vi "Configure Measurement (TOI - Tune Frequency).vi"(0 "VISA resource name":refnum<visa-resource-name>, 1 "Auto Upper Tune Frequency (T: Enable)":bool=TRUE, 2 "Manual Upper Tune Frequency  (2E+7 Hz)":dbl=20000000.0, 11 "error in (no error)":errorcluster, 12 "Auto Lower Tune Frequency (T: Enable)":bool=TRUE, 13 "Manual Lower Tune Frequency  (1E+7 Hz)":dbl=10000000.0) -> (4 "VISA resource name out":refnum<visa-resource-name>, 15 "error out":errorcluster)   [LabVIEW 2018, in "Agilent MXA Series.lvlib"]
doc: "Sets the TOI tune frequency measurement parameters."
uses:
  Agilent MXA Series.lvlib
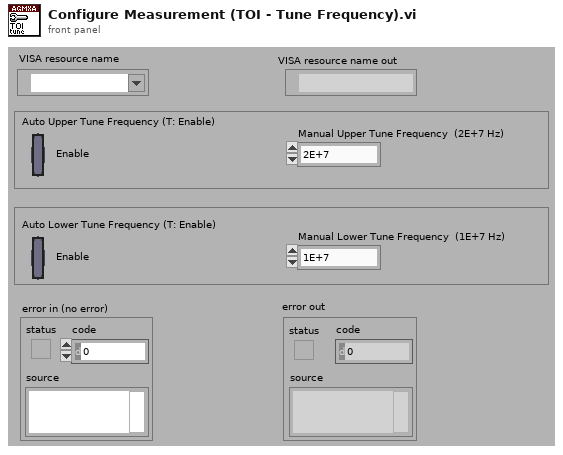
[diagram p1: front panel]
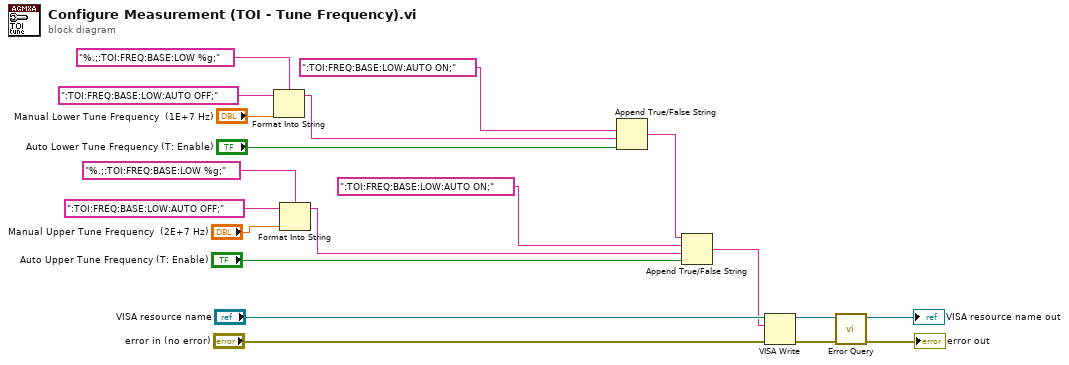
[diagram p0: block diagram]
diagram:
  n1 = Format Into String(format string="%.;:TOI:FREQ:BASE:LOW %g;", initial string=":TOI:FREQ:BASE:LOW:AUTO OFF;", "Manual Lower Tune Frequency  (1E+7 Hz)") -> (resulting string=w15:string)  [unwired: 1 in, 1 out]
  n2 = Format Into String(format string="%.;:TOI:FREQ:BASE:LOW %g;", initial string=":TOI:FREQ:BASE:LOW:AUTO OFF;", "Manual Upper Tune Frequency  (2E+7 Hz)") -> (resulting string=w4:string)  [unwired: 1 in, 1 out]
  n3 = Append True/False String(1:"Auto Lower Tune Frequency (T: Enable)", 2:w15, 3:":TOI:FREQ:BASE:LOW:AUTO ON;" ("true string")) -> (0:w2:string)  [unwired: 1 in]
  n4 = Append True/False String(1:"Auto Upper Tune Frequency (T: Enable)", 2:w4, 3:":TOI:FREQ:BASE:LOW:AUTO ON;" ("true string"), 4:w2) -> (0:w1:string)
  n5 = VISA Write(VISA resource name="VISA resource name", write buffer=w1, error in (no error)="error in (no error)") -> (VISA resource name out=w11:refnum<visa-resource-name>, error out=w12:errorcluster)  [unwired: 1 out]
  n6 = call "Error Query.vi"("error in (no error)"=w12, "VISA resource name"=w11) -> ("error out"=→"error out":errorcluster, "VISA resource name out"=→"VISA resource name out":refnum<visa-resource-name>)  [unwired: 6 in, 2 out]
